vi "TopLevel.vi"() -> ()   [LabVIEW 2020]
uses:
  Typedef.ctl
  TypeDefInLIb.ctl
  Lib.lvlib
panel:
  in  "Cluster 2":T1
  in  "Cluster":T2
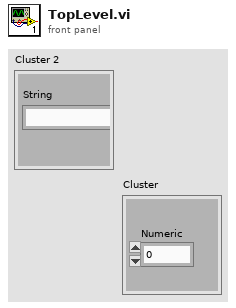
[diagram p1: front panel]
types:
  T1 = typedef "Lib.lvlib/TypeDefInLIb.ctl" = cluster{"String":string}
  T2 = typedef "Typedef.ctl" = cluster{"Numeric":dbl}
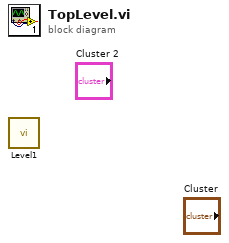
[diagram p0: block diagram]
diagram:
  n1 = call "Level1.vi"() -> ()  [unwired: 12 in]
